vi "OL.vi"(11 "CMD_OL":T1) -> (3 "OL CMD_OUT":T13={"Drive"={"CMDMODE"=enum."No Command", "X"=0.0, "Y"=0.0, "Rotation"=0.0, "Auto Angle"=0.0, "Speed Divider"=0.0, "Use Gyro"=FALSE, "Target Distance"=0.0}, "Hopper Feed"=0.0, "Shooter"={"Select"=enum."Manual VBus", "Wheel VBus"=0.0, "Wheel RPM"=0.0, "Hood VBus"=0.0, "Hood Position"=0.0}, "DONE"=FALSE, "Index"=0})   [LabVIEW 2017, in "Aim&ShootOverlord.lvlib"]
uses:
  Aim&ShootOverlord.lvlib
  ENUM_State.ctl
  ENUM_Action.ctl
  Cluster_OL Status.ctl
  Systems/MechamumDrive/Cluster_CMD to SM Data.ctl
  Systems/MechamumDrive/Enum_SM Cmd Select.ctl
  Systems/Shooter/Cluster_CMD to SM Data.ctl
  Systems/Shooter/ENUM_CMD Select.ctl
  Systems/Shooter/Cluster_SM Status.ctl
  Systems/MechamumDrive/Cluster_SM Status.ctl
  Systems/Shooter/Cluster_SM to HW Wheel Data.ctl
  Systems/Shooter/Cluster_SM to HW Hood Data.ctl
  Systems/MechamumDrive/Cluster_HW Status.ctl
  TypeDefs/Cluster_SRX Status With Encoder.ctl
  Systems/VisionSystem/Cluster_Vision Status.ctl
  Systems/VisionSystem/Enum_ Field Targets.ctl
  Cluster_CMD to OL Data.ctl
  Cluster_OL State Target.ctl
  Systems/Shooter/Global_SM_Data Out.vi
  Systems/MechamumDrive/Global_SM Out Data.vi
  Systems/MechamumDrive/Global_HW_Status Out.vi
  Systems/Sonar/Global_HW_Data Out.vi
  Systems/VisionSystem/Global_Vision Status.vi
  Systems/Shooter/Shooter.lvlib
  Systems/MechamumDrive/MechamunDrive.lvlib
  Systems/Sonar/Sonar.lvlib
  Systems/VisionSystem/VisionSystem.lvlib
panel:
  out "HW_Sonar Distance":dbl
  out "Vision Status":T4
  out "Drive_HW_Status":T6
  out "SM_Hood Data":T8
  out "SM_Wheel Data":T9
  out "Drive_SM_Status":T10
  out "Shooter SM_Status":T12
  out "Action":T17
  out "Current State":T3
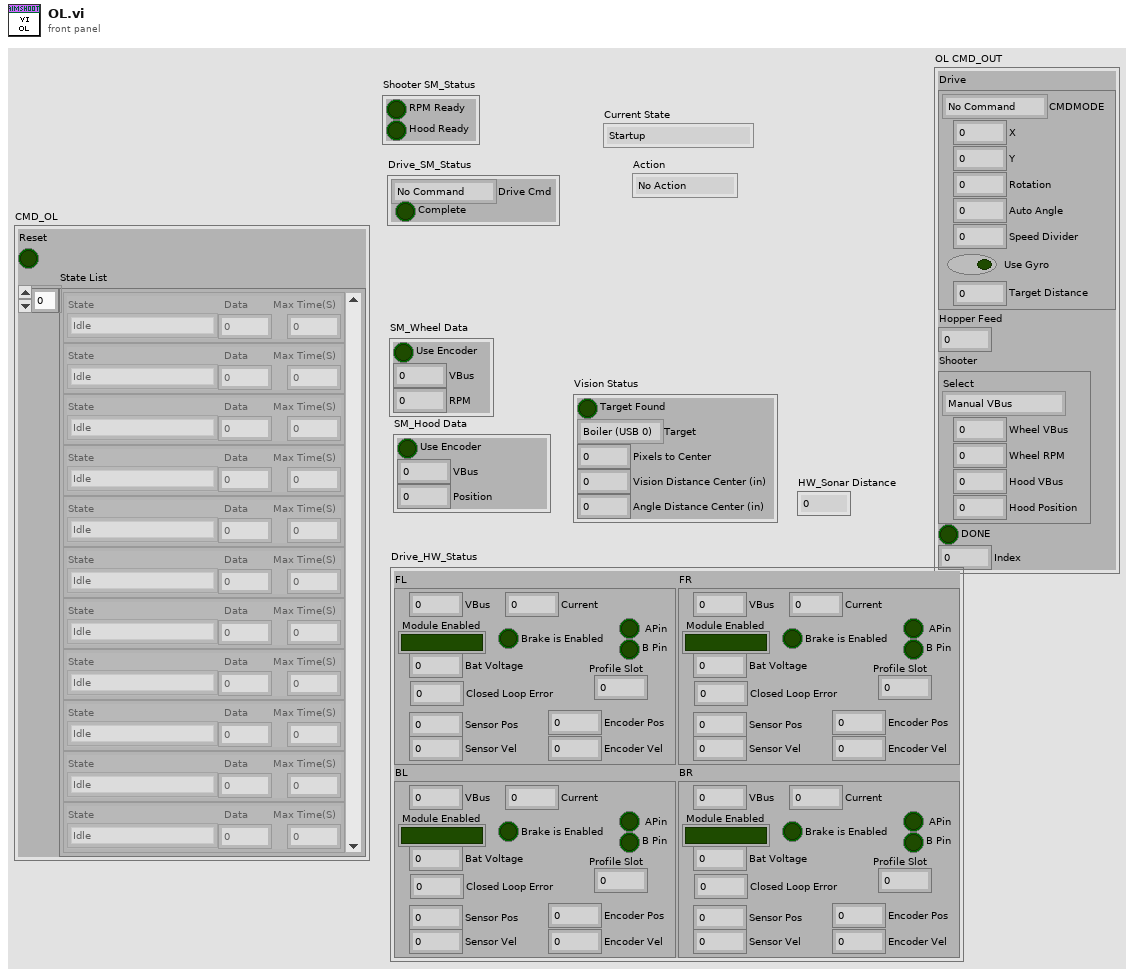
[diagram p1: front panel]
types:
  T1 = typedef "Aim&ShootOverlord.lvlib/Cluster_CMD to OL Data.ctl" = cluster{"Reset":bool, "State List":T2[]}
  T2 = typedef "Aim&ShootOverlord.lvlib/Cluster_OL State Target.ctl" = cluster{"State":T3, "Data":dbl, "Max Time(S)":dbl}
  T3 = typedef "Aim&ShootOverlord.lvlib/ENUM_State.ctl" = enum16{"Startup", "Idle", "Tracking Vis Rot", "Tracking Sonar Distance", "Waiting for Shooter", "Firing", "Timed Move", "Tracking Rotation", "Set State"}
  T4 = typedef "VisionSystem.lvlib/Cluster_Vision Status.ctl" = cluster{"Target Found":bool, "Target":T5, "Pixels to Center":dbl, "Vision Distance Center (in)":dbl, "Angle Distance Center (in)":dbl}
  T5 = typedef "VisionSystem.lvlib/Enum_ Field Targets.ctl" = enum16{"Boiler (USB 0)", "Rope (USB 1)"}
  T6 = typedef "MechamunDrive.lvlib/Cluster_HW Status.ctl" = cluster{"BL":T7, "BR":T7, "FL":T7, "FR":T7}
  T7 = typedef "Cluster_SRX Status With Encoder.ctl" = cluster{"VBus ":dbl, "Module Enabled":bool, "Closed Loop Error":dbl, "Sensor Pos":dbl, "Sensor Vel":dbl, "Current":dbl, "Brake is Enabled":bool, "Encoder Pos":dbl, "Encoder Vel":dbl, " APin":bool, "B Pin":bool, "Bat Voltage":dbl, "Profile Slot":dbl}
  T8 = typedef "Shooter.lvlib/Cluster_SM to HW Hood Data.ctl" = cluster{"Use Encoder":bool, "VBus":dbl, "Position":dbl}
  T9 = typedef "Shooter.lvlib/Cluster_SM to HW Wheel Data.ctl" = cluster{"Use Encoder":bool, "VBus":dbl, "RPM":dbl}
  T10 = typedef "MechamunDrive.lvlib/Cluster_SM Status.ctl" = cluster{"Drive Cmd":T11, "Complete":bool}
  T11 = typedef "MechamunDrive.lvlib/Enum_SM Cmd Select.ctl" = enum16{"No Command", "Halt", "Manual Keep Rotation", "Manual", "Track Front", "Track Rotation", "Track Lateral", "Track Vision Lat", "Track Vision Rot", "Strafe Right", "Strafe Left"}
  T12 = typedef "Shooter.lvlib/Cluster_SM Status.ctl" = cluster{"RPM Ready":bool, "Hood Ready":bool}
  T13 = typedef "Aim&ShootOverlord.lvlib/Cluster_OL Status.ctl" = cluster{"Drive":T14, "Hopper Feed":dbl, "Shooter":T15, "DONE":bool, "Index":i32}
  T14 = typedef "MechamunDrive.lvlib/Cluster_CMD to SM Data.ctl" = cluster{"CMDMODE":T11, "X":dbl, "Y":dbl, "Rotation":dbl, "Auto Angle":dbl, "Speed Divider":dbl, "Use Gyro":bool, "Target Distance":dbl}
  T15 = typedef "Shooter.lvlib/Cluster_CMD to SM Data.ctl" = cluster{"Select":T16, "Wheel VBus":dbl, "Wheel RPM":dbl, "Hood VBus":dbl, "Hood Position":dbl}
  T16 = typedef "Shooter.lvlib/ENUM_CMD Select.ctl" = enum16{"Stop", "Manual VBus", "Encoder Hood Only", "Encoder Wheel Only", "Encoder Both"}
  T17 = typedef "Aim&ShootOverlord.lvlib/ENUM_Action.ctl" = enum16{"No Action", "Reset Time", "Reset All", "Reset Index", "Increment Index", "Track Vis Rot", "Track Rotation", "Track Sonar", "Fire On", "Fire Off", "Shooter On", "Shooter Off", "Drive Stop", "Drive Forward"}
  T18 = cluster{"Yaw":dbl, "Roll":dbl, "Pitch":dbl, "Heading":dbl, "Fused Heading":dbl}
  T19 = cluster{"Actions":T17[], "State":T3, "Current Time":timestamp, "Start Time":timestamp, "CMD_OL":T1, "OL Status_OUT":T13, "SM_Wheel Data":T9, "SM_Hood Data":T8, "Shooter SM_Status":T12, "Drive_SM_Status":T10, "Drive_HW_Status":T6, "Vision Status":T4, "HW_Sonar Distance":dbl, "NavX":cluster{"Yaw":dbl, "Roll":dbl, "Pitch":dbl, "Heading":dbl, "Fused Heading":dbl}, "CMD_OL":T1, "Prev CMD_OL":T1}
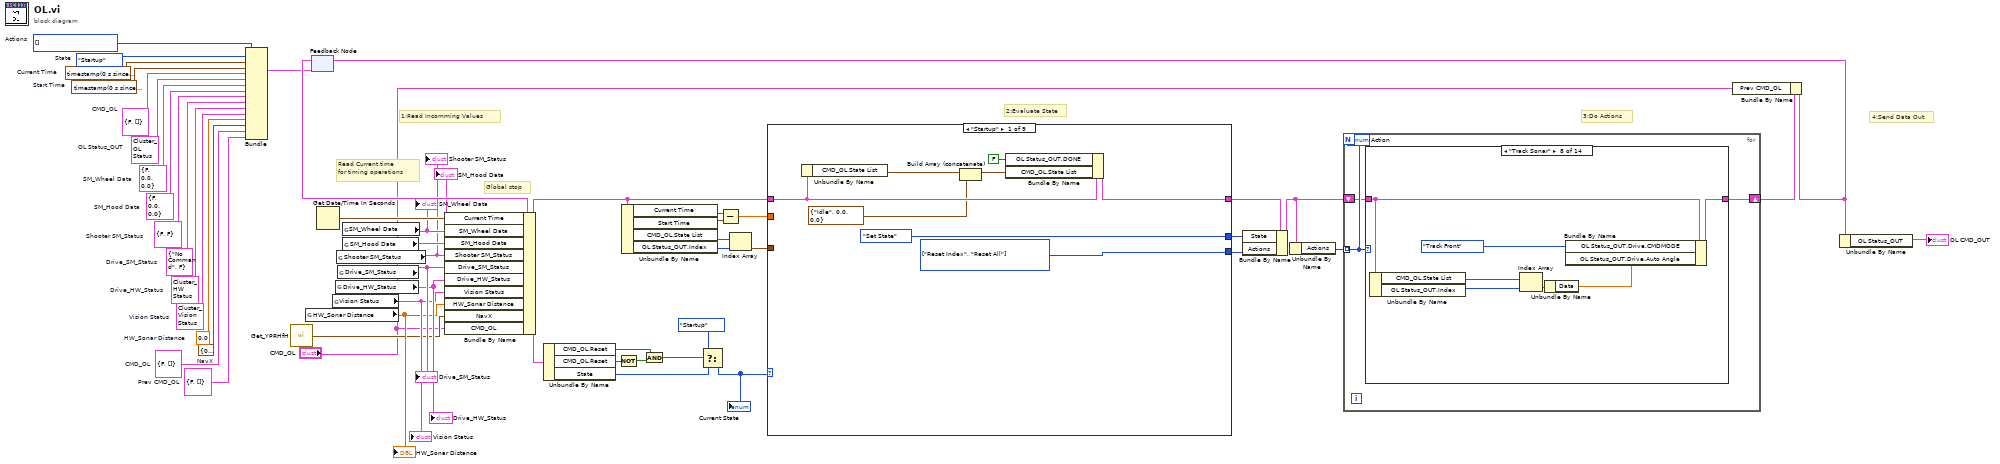
[diagram p0: block diagram]
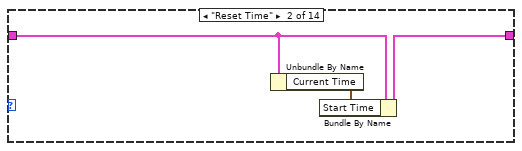
[diagram p3: hidden frame]
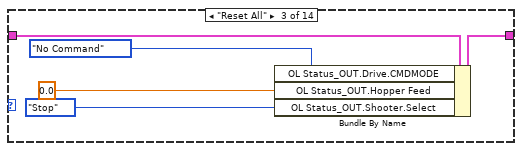
[diagram p4: hidden frame]
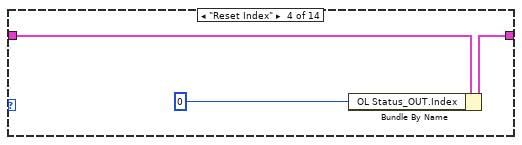
[diagram p5: hidden frame]
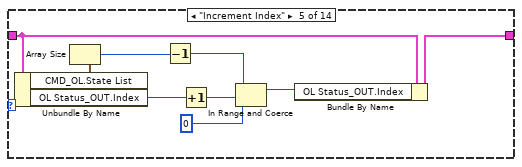
[diagram p6: hidden frame]
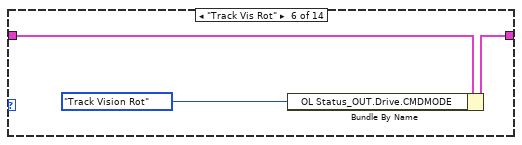
[diagram p7: hidden frame]
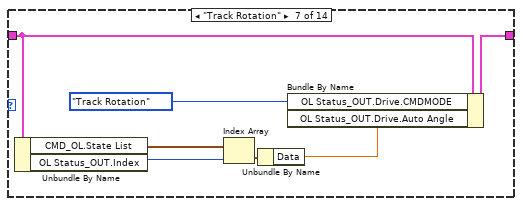
[diagram p8: hidden frame]
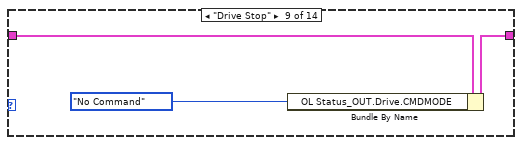
[diagram p9: hidden frame]
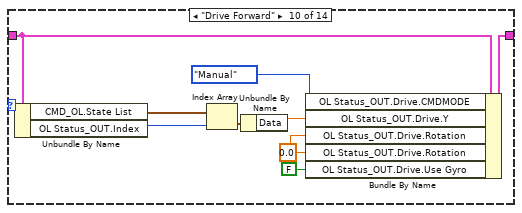
[diagram p10: hidden frame]
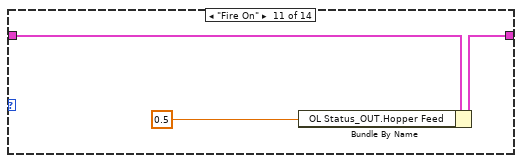
[diagram p11: hidden frame]
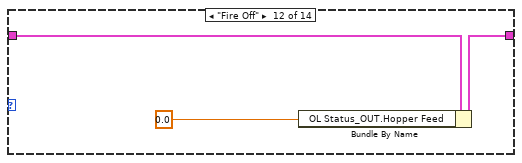
[diagram p12: hidden frame]
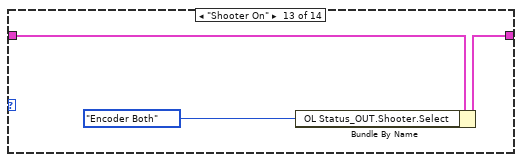
[diagram p13: hidden frame]
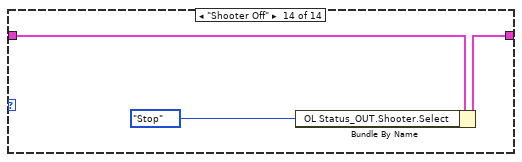
[diagram p14: hidden frame]
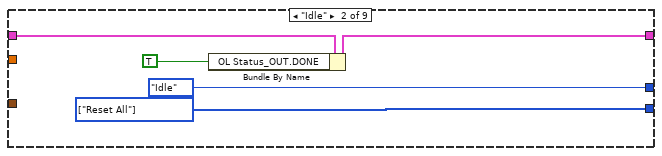
[diagram p15: hidden frame]
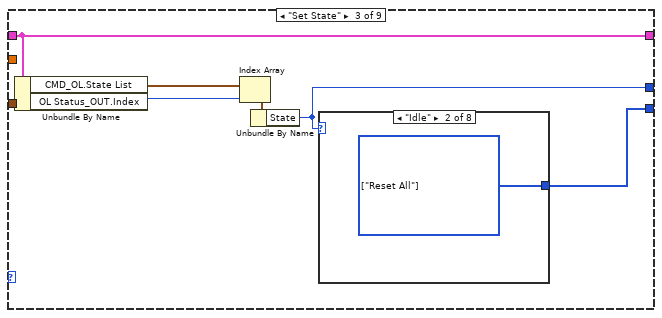
[diagram p16: hidden frame]
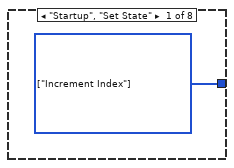
[diagram p17: hidden frame]
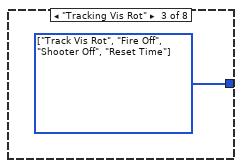
[diagram p18: hidden frame]
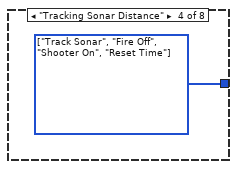
[diagram p19: hidden frame]
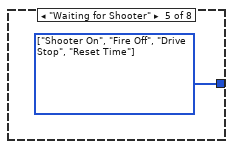
[diagram p20: hidden frame]
diagram:
  w8 = T1 {"Reset"=FALSE, "State List"=[]}  # CMD_OL
  w19 = T1 {"Reset"=FALSE, "State List"=[]}  # Prev CMD_OL
  w21 = T18 {"Yaw"=0.0, "Roll"=0.0, "Pitch"=0.0, "Heading"=0.0, "Fused Heading"=0.0}  # NavX
  w25 = 0.0  # HW_Sonar Distance
  w27 = T6 {"BL"={"VBus "=0.0, "Module Enabled"=FALSE, "Closed Loop Error"=0.0, "Sensor Pos"=0.0, "Sensor Vel"=0.0, "Current"=0.0, "Brake is Enabled"=FALSE, "Encoder Pos"=0.0, "Encoder Vel"=0.0, " APin"=FALSE, "B Pin"=FALSE, "Bat Voltage"=0.0, "Profile Slot"=0.0}, "BR"={"VBus "=0.0, "Module Enabled"=FALSE, "Closed Loop Error"=0.0, "Sensor Pos"=0.0, "Sensor Vel"=0.0, "Current"=0.0, "Brake is Enabled"=FALSE, "Encoder Pos"=0.0, "Encoder Vel"=0.0, " APin"=FALSE, "B Pin"=FALSE, "Bat Voltage"=0.0, "Profile Slot"=0.0}, "FL"={"VBus "=0.0, "Module Enabled"=FALSE, "Closed Loop Error"=0.0, "Sensor Pos"=0.0, "Sensor Vel"=0.0, "Current"=0.0, "Brake is Enabled"=FALSE, "Encoder Pos"=0.0, "Encoder Vel"=0.0, " APin"=FALSE, "B Pin"=FALSE, "Bat Voltage"=0.0, "Profile Slot"=0.0}, "FR"={"VBus "=0.0, "Module Enabled"=FALSE, "Closed Loop Error"=0.0, "Sensor Pos"=0.0, "Sensor Vel"=0.0, "Current"=0.0, "Brake is Enabled"=FALSE, "Encoder Pos"=0.0, "Encoder Vel"=0.0, " APin"=FALSE, "B Pin"=FALSE, "Bat Voltage"=0.0, "Profile Slot"=0.0}}  # Drive_HW_Status
  w26 = T4 {"Target Found"=FALSE, "Target"=enum."Boiler (USB 0)", "Pixels to Center"=0.0, "Vision Distance Center (in)"=0.0, "Angle Distance Center (in)"=0.0}  # Vision Status
  w29 = T10 {"Drive Cmd"=enum."No Command", "Complete"=FALSE}  # Drive_SM_Status
  w31 = T12 {"RPM Ready"=FALSE, "Hood Ready"=FALSE}  # Shooter SM_Status
  w33 = T8 {"Use Encoder"=FALSE, "VBus"=0.0, "Position"=0.0}  # SM_Hood Data
  w35 = T9 {"Use Encoder"=FALSE, "VBus"=0.0, "RPM"=0.0}  # SM_Wheel Data
  w45 = T13 {"Drive"={"CMDMODE"=enum."No Command", "X"=0.0, "Y"=0.0, "Rotation"=0.0, "Auto Angle"=0.0, "Speed Divider"=0.0, "Use Gyro"=FALSE, "Target Distance"=0.0}, "Hopper Feed"=0.0, "Shooter"={"Select"=enum."Manual VBus", "Wheel VBus"=0.0, "Wheel RPM"=0.0, "Hood VBus"=0.0, "Hood Position"=0.0}, "DONE"=FALSE, "Index"=0}  # OL Status_OUT
  w46 = T1 {"Reset"=FALSE, "State List"=[]}  # CMD_OL
  w47 = T17[] [] items=["No Action", "Reset Time", "Reset All", "Reset Index", "Increment Index", "Track Vis Rot", "Track Rotation", "Track Sonar", "Fire On", "Fire Off", "Shooter On", "Shooter Off", "Drive Stop", "Drive Forward"]  # Actions
  w48 = timestamp(0 s since 1904-01-01)  # Start Time
  w49 = timestamp(0 s since 1904-01-01)  # Current Time
  w50 = ENUM_State."Startup"  # State
  # "Read Current time\nfor timing operations"
  # "1:Read Incomming Values"
  # "2:Evaluate State"
  # "3:Do Actions"
  # "4:Send Data Out"
  # "Global stop"
  n1 = Bundle("Actions"=w47, "State"=w50, "Current Time"=w49, "Start Time"=w48, "CMD_OL"=w46, "OL Status_OUT"=w45, "SM_Wheel Data"=w35, "SM_Hood Data"=w33, "Shooter SM_Status"=w31, "Drive_SM_Status"=w29, "Drive_HW_Status"=w27, "Vision Status"=w26, "HW_Sonar Distance"=w25, "NavX"=w21, "CMD_OL"=w8, "Prev CMD_OL"=w19) -> (w43:T19)  [unwired: 1 in]
  n2 = call <vilib>:"Get_YPRHfH.vi"() -> ("YRPHfH"=w20:T18)  [unwired: 11 in]
  n3 = global read "Global_HW_Data Out.vi" "HW_Sonar Distance"() -> (w22:dbl)
  "HW_Sonar Distance" <- w22
  n4 = feedback #1(w43) -> (w44:T19)
  n5 = Get Date/Time In Seconds() -> (seconds since 1Jan1904=w41:timestamp)
  n6 = global read "Global_Vision Status.vi" "Vision Status"() -> (w23:T4)
  "Vision Status" <- w23
  n7 = global read "Global_HW_Status Out.vi" "Drive_HW_Status"() -> (w24:T6)
  "Drive_HW_Status" <- w24
  n8 = global read "Global_SM_Data Out.vi" "Shooter SM_Status"() -> (w30:T12)
  "Shooter SM_Status" <- w30
  n9 = global read "Global_SM Out Data.vi" "Drive_SM_Status"() -> (w28:T10)
  "Drive_SM_Status" <- w28
  n10 = global read "Global_SM_Data Out.vi" "SM_Wheel Data"() -> (w34:T9)
  "SM_Wheel Data" <- w34
  n11 = global read "Global_SM_Data Out.vi" "SM_Hood Data"() -> (w32:T8)
  "SM_Hood Data" <- w32
  n12 = Bundle By Name(cluster=w44, "Current Time"=w41, "SM_Wheel Data"=w34, "SM_Hood Data"=w32, "Shooter SM_Status"=w30, "Drive_SM_Status"=w28, "Drive_HW_Status"=w24, "Vision Status"=w23, "HW_Sonar Distance"=w22, "NavX"=w20, "CMD_OL"="CMD_OL") -> (w7:T19)
  n13 = Unbundle By Name(w7) -> ("CMD_OL.Reset"=w14:bool, "CMD_OL.Reset"=w16:bool, "State"=w11:T3)
  n14 = Not(x=w16) -> (.not. x?=w15:bool)
  n15 = Unbundle By Name(w7) -> ("Current Time"=w6:timestamp, "Start Time"=w5:timestamp, "CMD_OL.State List"=w3:T2[], "OL Status_OUT.Index"=w2:i32)
  n16 = And(x=w14, y=w15) -> (x .and. y?=w13:bool)
  n17 = Select(t=ENUM_State."Startup" ("Current State"), s=w13, f=w11) -> (s? t:f=w10:T3)
  "Current State" <- w10
  n18 = Subtract(x=w6, y=w5) -> (x-y=w4:dbl)
  n19 = Index Array(array=w3, index=w2) -> (element=w1:T2)
  n20 = case shown="\"Startup\"" w10 {
    selector: w10 -> [_ _ _ w82 w118 w154 w192 w203 w224]
    tunnel: w7 -> [w55 w61 w69 w80 w116 w152 w190 w201 w222]
    tunnel: [w56 w60 w69 w80 w116 w152 w190 w201 w222] -> w39
    tunnel: [ENUM_State."Set State" ("State") ENUM_State."Idle" ("State") w65 w79 w115 w151 w189 w200 w221] -> w38
    tunnel: [w57 w62 w64 w78 w114 w150 w188 w199 w220] -> w37
    tunnel: w4 -> [_ _ _ w83 w119 w155 w193 w204 w225]
    tunnel: w1 -> [_ _ _ w81 w117 w153 w191 w202 w223]
    frame "Startup" {
      w57 = T17[] [enum."Reset Index", enum."Reset All"] items=["No Action", "Reset Time", "Reset All", "Reset Index", "Increment Index", "Track Vis Rot", "Track Rotation", "Track Sonar", "Fire On", "Fire Off", "Shooter On", "Shooter Off", "Drive Stop", "Drive Forward"] ("Actions")
      n21 = Unbundle By Name(w55) -> ("CMD_OL.State List"=w54:T2[])
      n22 = Build Array (concatenate)(w54, T2 {"State"=enum."Idle", "Data"=0.0, "Max Time(S)"=0.0} ("OL State Target")) -> (w53:T2[])
      n23 = Bundle By Name(cluster=w55, "OL Status_OUT.DONE"=FALSE, "CMD_OL.State List"=w53) -> (w56:T19)
    }
    frame "Idle" {
      w62 = T17[] [enum."Reset All"] items=["No Action", "Reset Time", "Reset All", "Reset Index", "Increment Index", "Track Vis Rot", "Track Rotation", "Track Sonar", "Fire On", "Fire Off", "Shooter On", "Shooter Off", "Drive Stop", "Drive Forward"] ("Actions")
      n24 = Bundle By Name(cluster=w61, "OL Status_OUT.DONE"=TRUE) -> (w60:T19)
    }
    frame "Set State" {
      n25 = Unbundle By Name(w69) -> ("CMD_OL.State List"=w68:T2[], "OL Status_OUT.Index"=w67:i32)
      n26 = Index Array(array=w68, index=w67) -> (element=w66:T2)
      n27 = Unbundle By Name(w66) -> ("State"=w65:T3)
      n28 = case shown="\"Idle\"" w65 {
        tunnel: [w70 w71 w72 w73 w74 w75 w76 w77] -> w64
        frame "Startup", "Set State" {
          w70 = T17[] [enum."Increment Index"] items=["No Action", "Reset Time", "Reset All", "Reset Index", "Increment Index", "Track Vis Rot", "Track Rotation", "Track Sonar", "Fire On", "Fire Off", "Shooter On", "Shooter Off", "Drive Stop", "Drive Forward"] ("Actions")
        }
        frame "Idle" {
          w71 = T17[] [enum."Reset All"] items=["No Action", "Reset Time", "Reset All", "Reset Index", "Increment Index", "Track Vis Rot", "Track Rotation", "Track Sonar", "Fire On", "Fire Off", "Shooter On", "Shooter Off", "Drive Stop", "Drive Forward"] ("Actions")
        }
        frame "Tracking Vis Rot" {
          w72 = T17[] [enum."Track Vis Rot", enum."Fire Off", enum."Shooter Off", enum."Reset Time"] items=["No Action", "Reset Time", "Reset All", "Reset Index", "Increment Index", "Track Vis Rot", "Track Rotation", "Track Sonar", "Fire On", "Fire Off", "Shooter On", "Shooter Off", "Drive Stop", "Drive Forward"] ("Actions")
        }
        frame "Tracking Sonar Distance" {
          w73 = T17[] [enum."Track Sonar", enum."Fire Off", enum."Shooter On", enum."Reset Time"] items=["No Action", "Reset Time", "Reset All", "Reset Index", "Increment Index", "Track Vis Rot", "Track Rotation", "Track Sonar", "Fire On", "Fire Off", "Shooter On", "Shooter Off", "Drive Stop", "Drive Forward"] ("Actions")
        }
        frame "Waiting for Shooter" {
          w74 = T17[] [enum."Shooter On", enum."Fire Off", enum."Drive Stop", enum."Reset Time"] items=["No Action", "Reset Time", "Reset All", "Reset Index", "Increment Index", "Track Vis Rot", "Track Rotation", "Track Sonar", "Fire On", "Fire Off", "Shooter On", "Shooter Off", "Drive Stop", "Drive Forward"] ("Actions")
        }
        frame "Firing" {
          w75 = T17[] [enum."Shooter On", enum."Fire On", enum."Drive Stop", enum."Reset Time"] items=["No Action", "Reset Time", "Reset All", "Reset Index", "Increment Index", "Track Vis Rot", "Track Rotation", "Track Sonar", "Fire On", "Fire Off", "Shooter On", "Shooter Off", "Drive Stop", "Drive Forward"] ("Actions")
        }
        frame "Timed Move" {
          w76 = T17[] [enum."Drive Forward", enum."Reset Time", enum."Fire Off", enum."Shooter Off"] items=["No Action", "Reset Time", "Reset All", "Reset Index", "Increment Index", "Track Vis Rot", "Track Rotation", "Track Sonar", "Fire On", "Fire Off", "Shooter On", "Shooter Off", "Drive Stop", "Drive Forward"] ("Actions")
        }
        frame "Tracking Rotation" {
          w77 = T17[] [enum."Track Rotation", enum."Fire Off", enum."Shooter Off", enum."Reset Time"] items=["No Action", "Reset Time", "Reset All", "Reset Index", "Increment Index", "Track Vis Rot", "Track Rotation", "Track Sonar", "Fire On", "Fire Off", "Shooter On", "Shooter Off", "Drive Stop", "Drive Forward"] ("Actions")
        }
      }
    }
    frame "Tracking Vis Rot" {
      n29 = Unbundle By Name(w80) -> ("Drive_SM_Status.Drive Cmd"=w85:T11, "Drive_SM_Status.Complete"=w84:bool)
      n30 = case shown="\"Track Vision Rot\"" w85 {
        tunnel: w84 -> [w91 _]
        tunnel: w83 -> [w87 w107]
        tunnel: w82 -> [w86 w106]
        tunnel: w81 -> [w88 w108]
        tunnel: [w90 w110] -> w79
        tunnel: [w89 w109] -> w78
        frame "Track Vision Rot" {
          n31 = case shown="True" w91 {
            tunnel: [w94 ENUM_State."Set State" ("State")] -> w90
            tunnel: [w93 w102] -> w89
            tunnel: w88 -> [w98 _]
            tunnel: w87 -> [w97 _]
            tunnel: w86 -> [w92 _]
            frame False {
              n32 = Unbundle By Name(w98) -> ("Max Time(S)"=w96:dbl)
              n33 = Greater Or Equal?(x=w97, y=w96) -> (x >= y?=w95:bool)
              n34 = case shown="True" w95 {
                tunnel: [w99 ENUM_State."Set State" ("State")] -> w94
                tunnel: [_ w100] -> w93
                tunnel: w92 -> [w99 _]
                frame False {
                  # "Waiting for Complete"
                }
                frame True {
                  w100 = T17[] [enum."Increment Index", enum."Drive Stop"] items=["No Action", "Reset Time", "Reset All", "Reset Index", "Increment Index", "Track Vis Rot", "Track Rotation", "Track Sonar", "Fire On", "Fire Off", "Shooter On", "Shooter Off", "Drive Stop", "Drive Forward"] ("Actions")
                  # "Timeout"
                }
              }
            }
            frame True {
              w102 = T17[] [enum."Increment Index", enum."Drive Stop"] items=["No Action", "Reset Time", "Reset All", "Reset Index", "Increment Index", "Track Vis Rot", "Track Rotation", "Track Sonar", "Fire On", "Fire Off", "Shooter On", "Shooter Off", "Drive Stop", "Drive Forward"] ("Actions")
              # "Complete"
            }
          }
        }
        frame Default {
          n35 = Unbundle By Name(w108) -> ("Max Time(S)"=w105:dbl)
          n36 = Greater Or Equal?(x=w107, y=w105) -> (x >= y?=w104:bool)
          n37 = case shown="True" w104 {
            tunnel: [w111 ENUM_State."Set State" ("State")] -> w110
            tunnel: [_ w112] -> w109
            tunnel: w106 -> [w111 _]
            frame False {
              # "Waiting for Complete"
            }
            frame True {
              w112 = T17[] [enum."Increment Index", enum."Drive Stop"] items=["No Action", "Reset Time", "Reset All", "Reset Index", "Increment Index", "Track Vis Rot", "Track Rotation", "Track Sonar", "Fire On", "Fire Off", "Shooter On", "Shooter Off", "Drive Stop", "Drive Forward"] ("Actions")
              # "Timeout"
            }
          }
        }
      }
    }
    frame "Tracking Sonar Distance" {
      n38 = Unbundle By Name(w116) -> ("Drive_SM_Status.Drive Cmd"=w121:T11, "Drive_SM_Status.Complete"=w120:bool)
      n39 = case shown="\"Track Front\"" w121 {
        tunnel: w120 -> [w127 _]
        tunnel: w119 -> [w123 w143]
        tunnel: w118 -> [w122 w142]
        tunnel: w117 -> [w124 w144]
        tunnel: [w126 w146] -> w115
        tunnel: [w125 w145] -> w114
        frame "Track Front" {
          n40 = case shown="True" w127 {
            tunnel: [w130 ENUM_State."Set State" ("State")] -> w126
            tunnel: [w129 w138] -> w125
            tunnel: w124 -> [w134 _]
            tunnel: w123 -> [w133 _]
            tunnel: w122 -> [w128 _]
            frame False {
              n41 = Unbundle By Name(w134) -> ("Max Time(S)"=w132:dbl)
              n42 = Greater Or Equal?(x=w133, y=w132) -> (x >= y?=w131:bool)
              n43 = case shown="True" w131 {
                tunnel: [w135 ENUM_State."Set State" ("State")] -> w130
                tunnel: [_ w136] -> w129
                tunnel: w128 -> [w135 _]
                frame False {
                  # "Waiting for Complete"
                }
                frame True {
                  w136 = T17[] [enum."Increment Index", enum."Drive Stop"] items=["No Action", "Reset Time", "Reset All", "Reset Index", "Increment Index", "Track Vis Rot", "Track Rotation", "Track Sonar", "Fire On", "Fire Off", "Shooter On", "Shooter Off", "Drive Stop", "Drive Forward"] ("Actions")
                  # "Timeout"
                }
              }
            }
            frame True {
              w138 = T17[] [enum."Increment Index", enum."Drive Stop"] items=["No Action", "Reset Time", "Reset All", "Reset Index", "Increment Index", "Track Vis Rot", "Track Rotation", "Track Sonar", "Fire On", "Fire Off", "Shooter On", "Shooter Off", "Drive Stop", "Drive Forward"] ("Actions")
              # "Complete"
            }
          }
        }
        frame Default {
          n44 = Unbundle By Name(w144) -> ("Max Time(S)"=w141:dbl)
          n45 = Greater Or Equal?(x=w143, y=w141) -> (x >= y?=w140:bool)
          n46 = case shown="True" w140 {
            tunnel: [w147 ENUM_State."Set State" ("State")] -> w146
            tunnel: [_ w148] -> w145
            tunnel: w142 -> [w147 _]
            frame False {
              # "Waiting for Complete"
            }
            frame True {
              w148 = T17[] [enum."Increment Index", enum."Drive Stop"] items=["No Action", "Reset Time", "Reset All", "Reset Index", "Increment Index", "Track Vis Rot", "Track Rotation", "Track Sonar", "Fire On", "Fire Off", "Shooter On", "Shooter Off", "Drive Stop", "Drive Forward"] ("Actions")
              # "Timeout"
            }
          }
        }
      }
    }
    frame "Tracking Rotation" {
      n47 = Unbundle By Name(w152) -> ("Drive_SM_Status.Drive Cmd"=w157:T11, "Drive_SM_Status.Complete"=w156:bool)
      n48 = case shown="\"Track Rotation\"" w157 {
        tunnel: w156 -> [w163 _]
        tunnel: w155 -> [w159 w179]
        tunnel: w154 -> [w158 w178]
        tunnel: w153 -> [w160 w180]
        tunnel: [w162 w182] -> w151
        tunnel: [w161 w181] -> w150
        frame "Track Rotation" {
          n49 = case shown="False" w163 {
            tunnel: [w166 ENUM_State."Set State" ("State")] -> w162
            tunnel: [w165 w174] -> w161
            tunnel: w160 -> [w170 _]
            tunnel: w159 -> [w169 _]
            tunnel: w158 -> [w164 _]
            frame False {
              n50 = Unbundle By Name(w170) -> ("Max Time(S)"=w168:dbl)
              n51 = Greater Or Equal?(x=w169, y=w168) -> (x >= y?=w167:bool)
              n52 = case shown="True" w167 {
                tunnel: [w171 ENUM_State."Set State" ("State")] -> w166
                tunnel: [_ w172] -> w165
                tunnel: w164 -> [w171 _]
                frame False {
                  # "Waiting for Complete"
                }
                frame True {
                  w172 = T17[] [enum."Increment Index", enum."Drive Stop"] items=["No Action", "Reset Time", "Reset All", "Reset Index", "Increment Index", "Track Vis Rot", "Track Rotation", "Track Sonar", "Fire On", "Fire Off", "Shooter On", "Shooter Off", "Drive Stop", "Drive Forward"] ("Actions")
                  # "Timeout"
                }
              }
            }
            frame True {
              w174 = T17[] [enum."Increment Index", enum."Drive Stop"] items=["No Action", "Reset Time", "Reset All", "Reset Index", "Increment Index", "Track Vis Rot", "Track Rotation", "Track Sonar", "Fire On", "Fire Off", "Shooter On", "Shooter Off", "Drive Stop", "Drive Forward"] ("Actions")
              # "Complete"
            }
          }
        }
        frame Default {
          n53 = Unbundle By Name(w180) -> ("Max Time(S)"=w177:dbl)
          n54 = Greater Or Equal?(x=w179, y=w177) -> (x >= y?=w176:bool)
          n55 = case shown="True" w176 {
            tunnel: [w183 ENUM_State."Set State" ("State")] -> w182
            tunnel: [_ w184] -> w181
            tunnel: w178 -> [w183 _]
            frame False {
              # "Waiting for Complete"
            }
            frame True {
              w184 = T17[] [enum."Increment Index", enum."Drive Stop"] items=["No Action", "Reset Time", "Reset All", "Reset Index", "Increment Index", "Track Vis Rot", "Track Rotation", "Track Sonar", "Fire On", "Fire Off", "Shooter On", "Shooter Off", "Drive Stop", "Drive Forward"] ("Actions")
              # "Timeout"
            }
          }
        }
      }
    }
    frame "Timed Move" {
      n56 = Unbundle By Name(w191) -> ("Max Time(S)"=w187:dbl)
      n57 = Greater Or Equal?(x=w193, y=w187) -> (x >= y?=w186:bool)
      n58 = case shown="True" w186 {
        tunnel: [w194 ENUM_State."Set State" ("State")] -> w189
        tunnel: [_ w195] -> w188
        tunnel: w192 -> [w194 _]
        frame False {
          # "Waiting for Complete"
        }
        frame True {
          w195 = T17[] [enum."Increment Index", enum."Drive Stop"] items=["No Action", "Reset Time", "Reset All", "Reset Index", "Increment Index", "Track Vis Rot", "Track Rotation", "Track Sonar", "Fire On", "Fire Off", "Shooter On", "Shooter Off", "Drive Stop", "Drive Forward"] ("Actions")
          # "Complete"
        }
      }
    }
    frame "Waiting for Shooter" {
      n59 = Unbundle By Name(w201) -> ("Shooter SM_Status.Hood Ready"=w198:bool, "Shooter SM_Status.RPM Ready"=w205:bool)
      n60 = And(x=w198, y=w205) -> (x .and. y?=w197:bool)
      n61 = case shown="True" w197 {
        tunnel: w204 -> [w209 _]
        tunnel: w203 -> [w208 _]
        tunnel: w202 -> [w210 _]
        tunnel: [w212 ENUM_State."Set State" ("State")] -> w200
        tunnel: [w211 w216] -> w199
        frame False {
          n62 = Unbundle By Name(w210) -> ("Max Time(S)"=w207:dbl)
          n63 = Greater Or Equal?(x=w209, y=w207) -> (x >= y?=w206:bool)
          n64 = case shown="True" w206 {
            tunnel: [w213 ENUM_State."Set State" ("State")] -> w212
            tunnel: [_ w214] -> w211
            tunnel: w208 -> [w213 _]
            frame False {
              # "Waiting for Complete"
            }
            frame True {
              w214 = T17[] [enum."Increment Index"] items=["No Action", "Reset Time", "Reset All", "Reset Index", "Increment Index", "Track Vis Rot", "Track Rotation", "Track Sonar", "Fire On", "Fire Off", "Shooter On", "Shooter Off", "Drive Stop", "Drive Forward"] ("Actions")
              # "Timeout"
            }
          }
        }
        frame True {
          w216 = T17[] [enum."Increment Index"] items=["No Action", "Reset Time", "Reset All", "Reset Index", "Increment Index", "Track Vis Rot", "Track Rotation", "Track Sonar", "Fire On", "Fire Off", "Shooter On", "Shooter Off", "Drive Stop", "Drive Forward"] ("Actions")
          # "Complete"
        }
      }
    }
    frame "Firing" {
      n65 = Unbundle By Name(w223) -> ("Max Time(S)"=w219:dbl)
      n66 = Greater Or Equal?(x=w225, y=w219) -> (x >= y?=w218:bool)
      n67 = case shown="False" w218 {
        tunnel: [w226 ENUM_State."Set State" ("State")] -> w221
        tunnel: [_ w227] -> w220
        tunnel: w224 -> [w226 _]
        frame False {
          # "Waiting for Complete"
        }
        frame True {
          w227 = T17[] [enum."Increment Index"] items=["No Action", "Reset Time", "Reset All", "Reset Index", "Increment Index", "Track Vis Rot", "Track Rotation", "Track Sonar", "Fire On", "Fire Off", "Shooter On", "Shooter Off", "Drive Stop", "Drive Forward"] ("Actions")
          # "Complete"
        }
      }
    }
  }
  n68 = Bundle By Name(cluster=w39, "State"=w38, "Actions"=w37) -> (w40:T19)
  n69 = Unbundle By Name(w40) -> ("Actions"=w42:T17[])
  n70 = for {
    tunnel: w42 -> [w231] mode=indexing
    shift-right: [w230] -> w18
    shift-left: w40 -> [w229]
    n71 = case shown="\"Track Sonar\"" w231 {
      tunnel: w229 -> [w232 w235 w240 w243 w251 w255 w260 w267 w270 w279 w283 w286 w289 w292]
      tunnel: [w232 w234 w239 w242 w252 w254 w262 w269 w272 w281 w284 w287 w290 w293] -> w230
      frame "No Action" {
      }
      frame "Reset Time" {
        n72 = Unbundle By Name(w235) -> ("Current Time"=w233:timestamp)
        n73 = Bundle By Name(cluster=w235, "Start Time"=w233) -> (w234:T19)
      }
      frame "Reset All" {
        n74 = Bundle By Name(cluster=w240, "OL Status_OUT.Drive.CMDMODE"=Enum_SM_Cmd_Select."No Command", "OL Status_OUT.Hopper Feed"=0.0, "OL Status_OUT.Shooter.Select"=ENUM_CMD_Select."Stop") -> (w239:T19)
      }
      frame "Reset Index" {
        n75 = Bundle By Name(cluster=w243, "OL Status_OUT.Index"=0 ("Index")) -> (w242:T19)
      }
      frame "Increment Index" {
        n76 = Unbundle By Name(w251) -> ("CMD_OL.State List"=w250:T2[], "OL Status_OUT.Index"=w248:i32)
        n77 = Array Size(array=w250) -> (size(s)=w249:i32)
        n78 = Decrement(x=w249) -> (x-1=w246:i32)
        n79 = Increment(x=w248) -> (x+1=w247:i32)
        n80 = In Range and Coerce(upper limit=w246, x=w247, lower limit=0) -> (coerced(x)=w245:i32)  [unwired: 1 out]
        n81 = Bundle By Name(cluster=w251, "OL Status_OUT.Index"=w245) -> (w252:T19)
      }
      frame "Track Vis Rot" {
        n82 = Bundle By Name(cluster=w255, "OL Status_OUT.Drive.CMDMODE"=Enum_SM_Cmd_Select."Track Vision Rot") -> (w254:T19)
      }
      frame "Track Rotation" {
        n83 = Unbundle By Name(w260) -> ("CMD_OL.State List"=w259:T2[], "OL Status_OUT.Index"=w258:i32)
        n84 = Index Array(array=w259, index=w258) -> (element=w257:T2)
        n85 = Unbundle By Name(w257) -> ("Data"=w256:dbl)
        n86 = Bundle By Name(cluster=w260, "OL Status_OUT.Drive.CMDMODE"=Enum_SM_Cmd_Select."Track Rotation", "OL Status_OUT.Drive.Auto Angle"=w256) -> (w262:T19)
      }
      frame "Track Sonar" {
        n87 = Unbundle By Name(w267) -> ("CMD_OL.State List"=w266:T2[], "OL Status_OUT.Index"=w265:i32)
        n88 = Index Array(array=w266, index=w265) -> (element=w264:T2)
        n89 = Unbundle By Name(w264) -> ("Data"=w263:dbl)
        n90 = Bundle By Name(cluster=w267, "OL Status_OUT.Drive.CMDMODE"=Enum_SM_Cmd_Select."Track Front", "OL Status_OUT.Drive.Auto Angle"=w263) -> (w269:T19)
      }
      frame "Drive Stop" {
        n91 = Bundle By Name(cluster=w270, "OL Status_OUT.Drive.CMDMODE"=Enum_SM_Cmd_Select."No Command") -> (w272:T19)
      }
      frame "Drive Forward" {
        w273 = 0.0 ("OL Status_OUT.Drive.Rotation")
        n92 = Unbundle By Name(w279) -> ("CMD_OL.State List"=w278:T2[], "OL Status_OUT.Index"=w277:i32)
        n93 = Index Array(array=w278, index=w277) -> (element=w276:T2)
        n94 = Unbundle By Name(w276) -> ("Data"=w275:dbl)
        n95 = Bundle By Name(cluster=w279, "OL Status_OUT.Drive.CMDMODE"=Enum_SM_Cmd_Select."Manual", "OL Status_OUT.Drive.Y"=w275, "OL Status_OUT.Drive.Rotation"=w273, "OL Status_OUT.Drive.Rotation"=w273, "OL Status_OUT.Drive.Use Gyro"=FALSE) -> (w281:T19)
      }
      frame "Fire On" {
        n96 = Bundle By Name(cluster=w283, "OL Status_OUT.Hopper Feed"=0.5) -> (w284:T19)
      }
      frame "Fire Off" {
        n97 = Bundle By Name(cluster=w286, "OL Status_OUT.Hopper Feed"=0.0) -> (w287:T19)
      }
      frame "Shooter On" {
        n98 = Bundle By Name(cluster=w289, "OL Status_OUT.Shooter.Select"=ENUM_CMD_Select."Encoder Both") -> (w290:T19)
      }
      frame "Shooter Off" {
        n99 = Bundle By Name(cluster=w292, "OL Status_OUT.Shooter.Select"=ENUM_CMD_Select."Stop") -> (w293:T19)
      }
    }
    "Action" <- w231
  }
  n100 = Bundle By Name(cluster=w18, "Prev CMD_OL"="CMD_OL") -> (w17:T19)
  n101 = feedback-in #1(w17) -> ()
  n102 = Unbundle By Name(w17) -> ("OL Status_OUT"=→"OL CMD_OUT":T13)
